vi "CMD_CLEARLOG.vi"(7 "Console Log in":refnum<class "Console Log.lvclass">, 8 "error in (no error)":errorcluster, 10 "Arguments":string[](array[string]), 11 "gScript Interpreter in":refnum<class "gScript Interpreter.lvclass">) -> (0 "error out":errorcluster, 3 "gScript Interpreter out":refnum<class "gScript Interpreter.lvclass">, 5 "Console Log out":refnum<class "Console Log.lvclass">)   [LabVIEW 2023, in "gScript Interpreter.lvclass"]
uses:
  gScript Interpreter.lvclass
  Application Utilities/Console Log/Console Log.lvclass
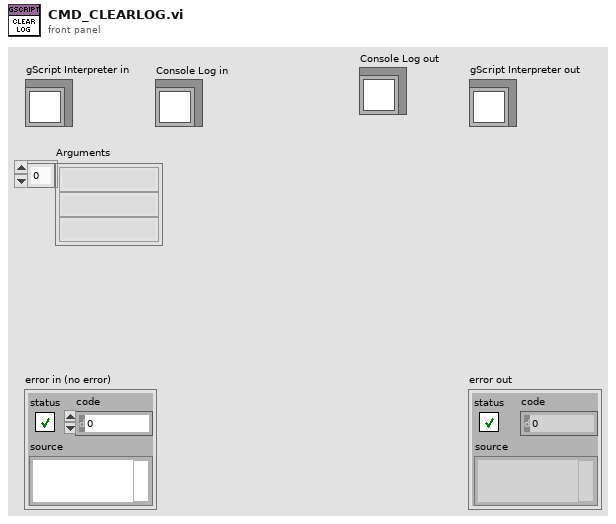
[diagram p1: front panel]
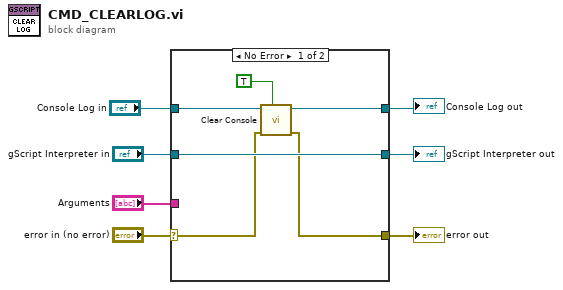
[diagram p0: block diagram]
diagram:
  n1 = case shown="No Error" "error in (no error)" {
    selector: "error in (no error)" -> [w10 w16]
    tunnel: [w9 w16] -> w6
    tunnel: [w13 w15] -> w4
    tunnel: "gScript Interpreter in" -> [w13 w15]
    tunnel: "Arguments" -> [_ _]
    tunnel: "Console Log in" -> [w12 w14]
    tunnel: [w11 w14] -> w1
    frame No Error {
      n2 = call "Clear Console.vi"("Clear Logfile"=TRUE, "error in (no error)"=w10, "Console Log in"=w12) -> ("error out"=w9:errorcluster, "Console Log out"=w11:refnum<class "Console Log.lvclass">)  [unwired: 7 in]
    }
    frame Error {
    }
  }
  "error out" <- w6
  "gScript Interpreter out" <- w4
  "Console Log out" <- w1
